vi "Waveform Cluster (1D) to Spreadsheet String.vi"(1 "waveform cluster":cluster{i32, "dx":dbl, "Array":dbl[]}) -> (0 "spreadsheet string":string)   [LabVIEW 2015]
uses:
  Math VIs/LinSpace (x0-dx-npts).vi
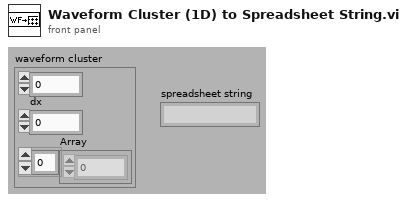
[diagram p1: front panel]
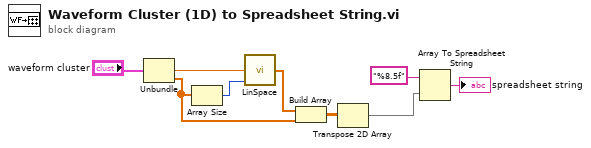
[diagram p0: block diagram]
diagram:
  n1 = Unbundle("waveform cluster") -> ("dx"=w8:dbl, "Array"=w4:dbl[])  [unwired: 1 out]
  n2 = Array Size(array=w4) -> (size(s)=w7:i32)
  n3 = call-poly "LinSpace.vi"("npts"=w7, "dx"=w8) -> ("Array"=w5:dbl[])  [unwired: 2 in, 1 out]
  n4 = Build Array(w5, w4) -> (w3:dbl[][])
  n5 = Transpose 2D Array(2D array=w3) -> (transposed array=w2:dbl[][])
  n6 = Array To Spreadsheet String(array=w2, 3:"%8.5f" ("format (%.3f)")) -> (spreadsheet string=→"spreadsheet string":string)  [unwired: 1 in]
